vi "Curtin1_ClearPlots.vi"(11 "Array":refnum<vi>[](array[refnum])) -> ()   [LabVIEW 2022 SP3]
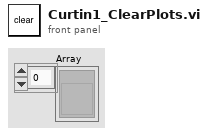
[diagram p1: front panel]
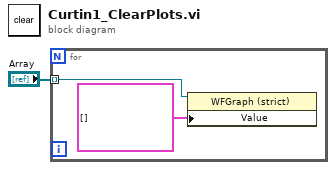
[diagram p0: block diagram]
diagram:
  n1 = for {
    tunnel: "Array" -> [w3] mode=indexing
    n2 = property class="WFGraph (strict)"(reference=w3, "Value"=cluster{dbl, "df":dbl, dbl[]}[] []) -> ()  [unwired: 1 in, 2 out]
  }
